vi "Detect edge angles.vi"(0 "Image filepath":path=path "E:/Algorithm/Geometric template matching/Images/Partially symmetric part/2.png", 1 "Auto ROI detect":bool=TRUE, 2 "Remove dust?":bool=TRUE, 3 "ROI parameters\nFeature":T5={"Step Size"=500, "r offset"=500, "Edge Options"={"Edge Polarity"=0, "Kernel Size"=5, "Width"=3, "Minimum Edge Strength"=120.0, "Interpolation Type"=enum."Bilinear Fixed", "Data Processing Method"=enum."Average"}, "Annulus\ndetails"={"Center X"=0, "Center Y"=0, "Inner Radius"=10, "Outer Radius"=4000, "Start Angle"=0.0, "End Angle"=0.0}} {"Edge Options"."Edge Polarity" items=["All Edges", "Rising Edges", "Falling Edges"]; "Edge Options"."Minimum Edge Strength" format="%.2f"; "Edge Options"."Width" step=2; "Edge Options"."Kernel Size" step=2; "Annulus\ndetails"."End Angle" min=-90.0 max=90.0 step=1.0 format="%.2f"; "Annulus\ndetails"."Start Angle" min=-90.0 max=90.0 step=1.0 format="%.2f"; "Annulus\ndetails"."Center X" scale=0.0..1024.0}, 4 "Image input?":bool, 5 "error in":errorcluster, 6 "Image in":T1, 7 "Overlay?":bool=TRUE, 8 "Dispose\nimage?":bool, 9 "Dust removal data":T7={"Dilate data"={"Operation"=enum."Erode", "Structuring Element"=[[1, 1, 1], [1, 1, 1], [1, 1, 1]], "Number of iterations (1)"=1, "Square/Hexa (Square)"=TRUE}, "Threshold data"={"Method (clustering)"=0, "Look For (Bright Objects)"=1, "Range"={"Lower value"=128.0, "Upper value"=255.0}, "Replace Value"=1.0}} {"Threshold data"."Look For (Bright Objects)" items=["Bright Objects", "Dark Objects"]; "Threshold data"."Method (clustering)" items=["clustering", "entropy", "metric", "moments", "inter-class variance"]}, 11 "BufferData":cluster{"Image Name":string}={"Image Name"="LearnTempImage"}) -> (10 "ROI parameters\nFeature out":T8 {"Edge Options"."Edge Polarity" items=["All Edges", "Rising Edges", "Falling Edges"]; "Edge Options"."Minimum Edge Strength" format="%.2f"; "Edge Options"."Width" step=2; "Edge Options"."Kernel Size" step=2; "Annulus\ndetails"."End Angle" min=-90.0 max=90.0 step=1.0 format="%.2f"; "Annulus\ndetails"."Start Angle" min=-90.0 max=90.0 step=1.0 format="%.2f"; "Annulus\ndetails"."Center X" scale=0.0..1024.0}, 14 "Output":T6, 16 "Image indicator":T1(plugin-control), 19 "error out":errorcluster)   [LabVIEW 2019]
uses:
  <vilib>/vision/Image Controls.llb/IMAQ Image.ctl
  <vilib>/vision/Measure.llb/Edge Options.ctl
  <vilib>/vision/Measure.llb/Edge Polarity.ctl
  <vilib>/Utility/file.llb/Write Delimited Spreadsheet (DBL).vi
  Controls/ROI parameters.ctl
panel:
  in  "Tab Control":enum32{"Display image", "Misc."}(tab)
  out "Output filepath":path
  in  "stop":bool
  out "Cycle time (in seconds)":dbl
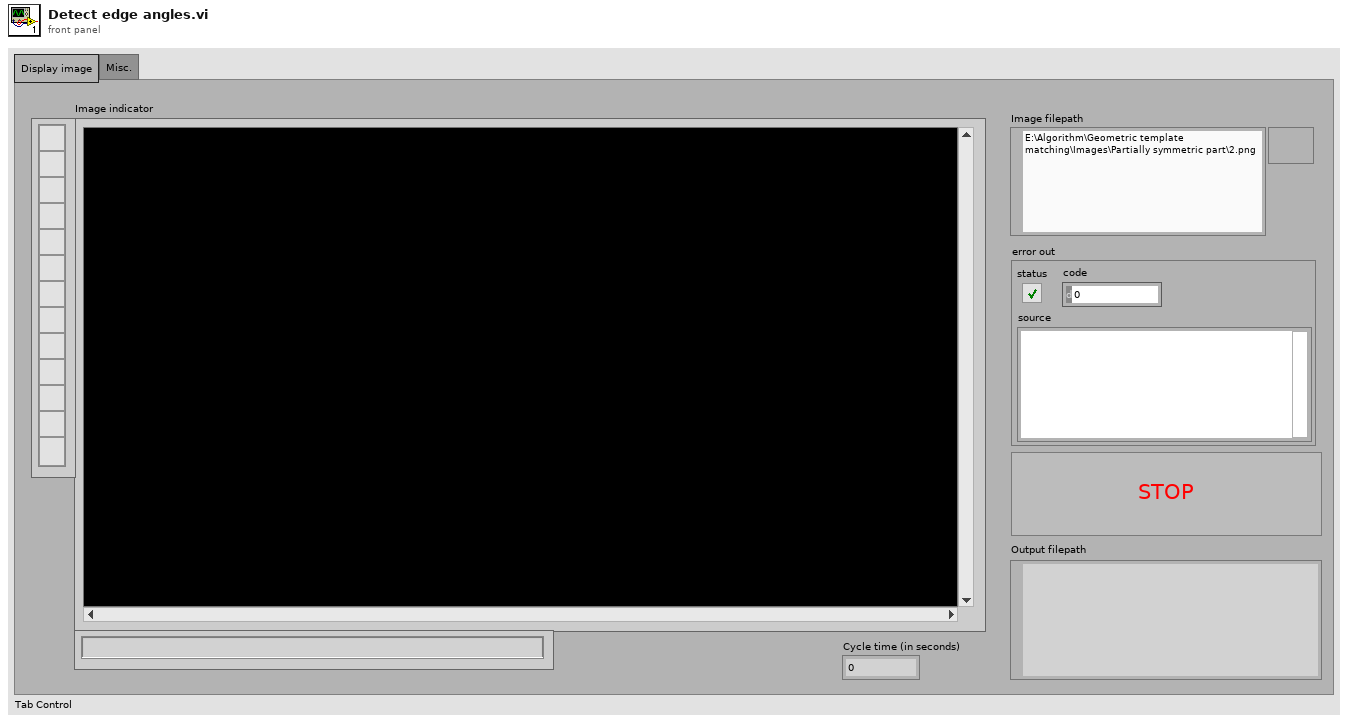
[diagram p1: front panel]
types:
  T1 = typedef "IMAQ Image.ctl" = refnum<image>
  T2 = typedef "Edge Options.ctl" = cluster{"Edge Polarity":T3, "Kernel Size":u32, "Width":u32, "Minimum Edge Strength":sgl, "Interpolation Type":enum32{"Zero Order", "Bilinear", "Quadratic", "Cubic", "Bilinear Fixed"}, "Data Processing Method":enum32{"Average", "Median"}}
  T3 = typedef "Edge Polarity.ctl" = u32
  T4 = typedef "IMAQ Circle" = cluster{"Center X":i32, "Center Y":i32, "Inner Radius":i32, "Outer Radius":i32, "Start Angle":dbl, "End Angle":dbl}
  T5 = cluster{"Step Size":u32, "r offset":u32, "Edge Options":T2, "Annulus\ndetails":T4}
  T6 = cluster{"Angle info":cluster{"Rising edge angles":cluster{"Edge angles":dbl[]}[], "Falling edge angles":cluster{"Edge angles":dbl[]}[]}, "Center":cluster{"X":sgl, "Y":sgl}}
  T7 = cluster{"Dilate data":cluster{"Operation":enum32{"AutoM", "Close", "Dilate", "Erode", "Gradient", "Gradient out", "Gradient in", "Hit miss", "Open", "PClose", "POpen", "Thick", "Thin"}, "Structuring Element":i32[][], "Number of iterations (1)":i32, "Square/Hexa (Square)":bool}, "Threshold data":cluster{"Method (clustering)":i32, "Look For (Bright Objects)":u32, "Range":cluster{"Lower value":sgl, "Upper value":sgl}, "Replace Value":sgl}}
  T8 = typedef "ROI parameters.ctl" = cluster{"Step Size":u32, "r offset":u32, "Edge Options":T2, "Annulus\ndetails":T4}
  T9 = cluster{"Rising edge angles":cluster{"Edge angles":dbl[]}[], "Falling edge angles":cluster{"Edge angles":dbl[]}[]}
  T10 = cluster{"Edges (Rising)":cluster{"Location":cluster{"X":sgl, "Y":sgl}[]}[], "Edges (Falling)":cluster{"Location":cluster{"X":sgl, "Y":sgl}[]}[], "ROI parameters\nFeature.Edge Options":T2}
  T11 = cluster{"Global Rectangle":i32[], "Contours":cluster{"Contour Type":u32, "ROI Type":u32, "Points":i32[]}[]}
  T12 = cluster{"Center":cluster{"X":sgl, "Y":sgl}, "Radius":dbl}
  T13 = cluster{"Edge ROI":cluster{"Global Rectangle":i32[], "Contours":cluster{"Contour Type":u32, "ROI Type":u32, "Points":i32[]}[]}, "Previous state":string, "Circle 1 detaiils":cluster{"Center":cluster{"X":sgl, "Y":sgl}, "Radius":dbl}, "Image indicator":refnum<vi>, "Image \narray":T1[], "Edge point location":cluster{"X":sgl, "Y":sgl}[], "Angles":sgl[], "Output filename":string, "Tick count (Start)":u32, "ROI parameters\nFeature":cluster{"Step Size":u32, "r offset":u32, "Edge Options":T2, "Annulus\ndetails":T4}, "Edge info":cluster{"Edges (Rising)":cluster{"Location":cluster{"X":sgl, "Y":sgl}[]}[], "Edges (Falling)":cluster{"Location":cluster{"X":sgl, "Y":sgl}[]}[], "ROI parameters\nFeature.Edge Options":T2}, "Angle info":cluster{"Rising edge angles":cluster{"Edge angles":dbl[]}[], "Falling edge angles":cluster{"Edge angles":dbl[]}[]}, "Dust removal data":cluster{"Dilate data":cluster{"Operation":enum32{"AutoM", "Close", "Dilate", "Erode", "Gradient", "Gradient out", "Gradient in", "Hit miss", "Open", "PClose", "POpen", "Thick", "Thin"}, "Structuring Element":i32[][], "Number of iterations (1)":i32, "Square/Hexa (Square)":bool}, "Threshold data":cluster{"Method (clustering)":i32, "Look For (Bright Objects)":u32, "Range":cluster{"Lower value":sgl, "Upper value":sgl}, "Replace Value":sgl}}, "Remove dust?":bool, "Auto ROI detect":bool, "Image size factor":dbl, "Image in":T1, "Overlay?":bool, "BufferData":cluster{"Image Name":string}}
  T14 = cluster{"Objects":u16, "Threshold":i32, "Reject Border":bool, "Fill Holes":bool, "Min Object Size":bool, "Min Size":i32, "Max Object Size":bool, "Max Size":i32, "Show Search Area":bool, "Show Center":bool, "Show Bounding Box":bool}
  T15 = typedef "ROI Descriptor" = cluster{"Global Rectangle":i32[], "Contours":cluster{"ID":enum32{"External", "Internal"}, "Type":u32, "Coordinates":i32[]}[]}
  T16 = cluster{"Object Center":cluster{"X":sgl, "Y":sgl}, "Bounding Box":cluster{"X Left":i32, "Y Top":i32, "X Right":i32, "Y Bottom":i32}, "Area":sgl, "Orientation":sgl, "Aspect Ratio":sgl, "Nb Holes":i32}[]
  T17 = cluster{"Object Center":cluster{"X":sgl, "Y":sgl}, "Bounding Box":cluster{"X Left":i32, "Y Top":i32, "X Right":i32, "Y Bottom":i32}, "Area":sgl, "Orientation":sgl, "Aspect Ratio":sgl, "Nb Holes":i32}
  T18 = cluster{"Location":cluster{"X":sgl, "Y":sgl}[]}[]
  T19 = typedef "Image Type" = u32
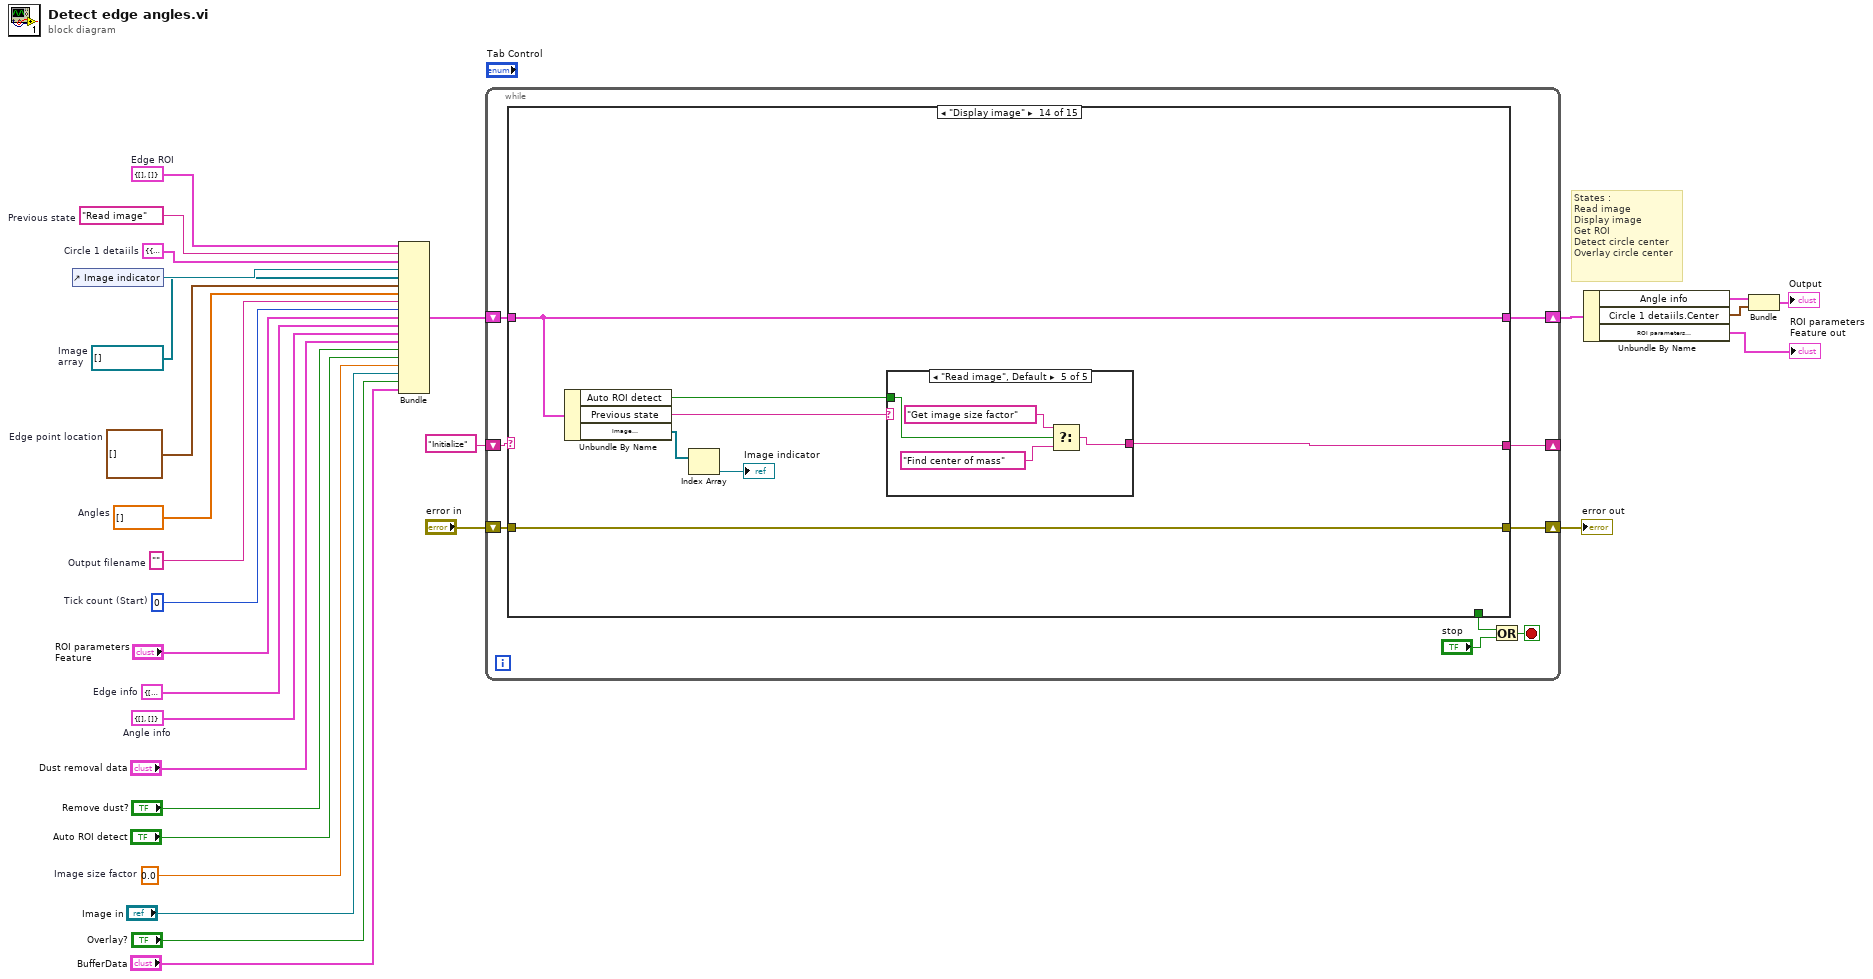
[diagram p0: block diagram]
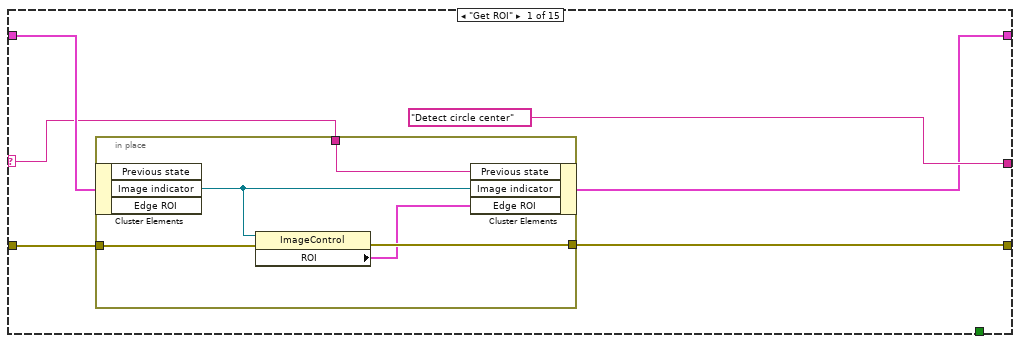
[diagram p2: hidden frame]
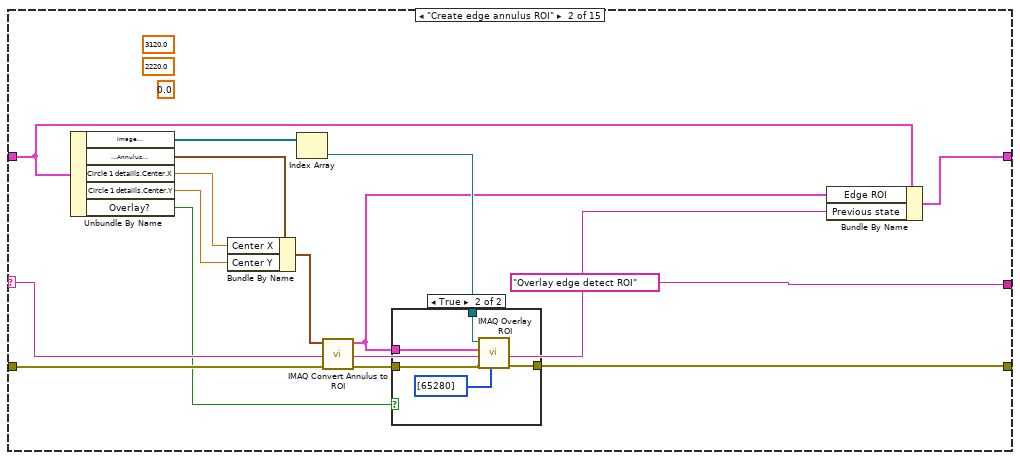
[diagram p3: hidden frame]
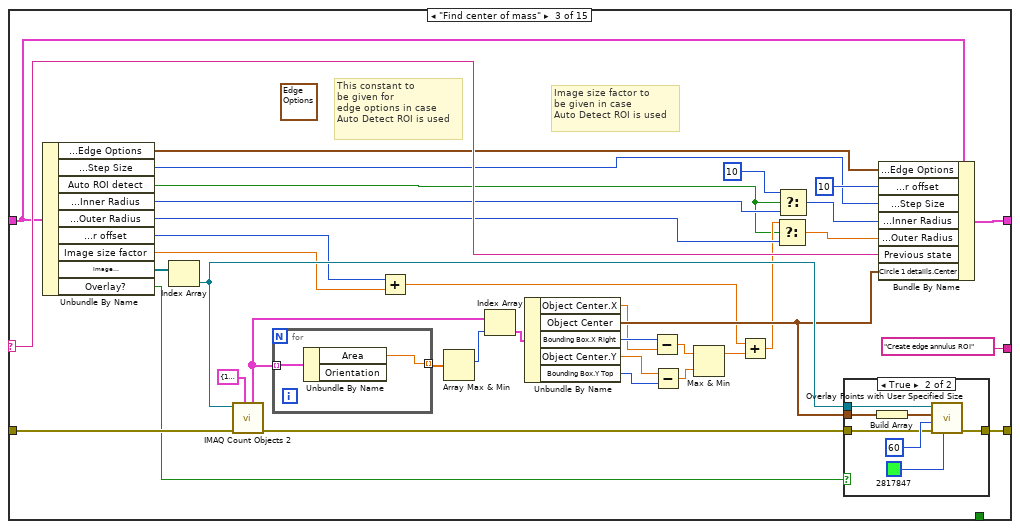
[diagram p5: hidden frame]
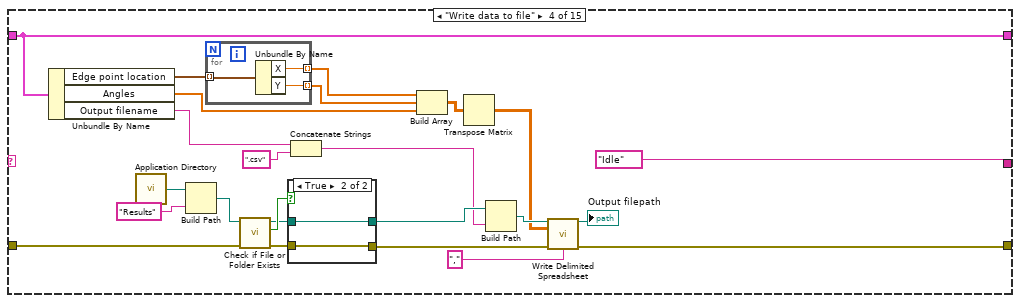
[diagram p7: hidden frame]
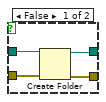
[diagram p8: hidden frame]
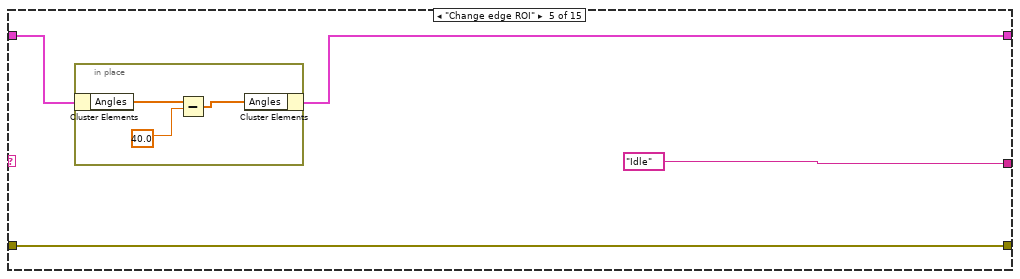
[diagram p9: hidden frame]
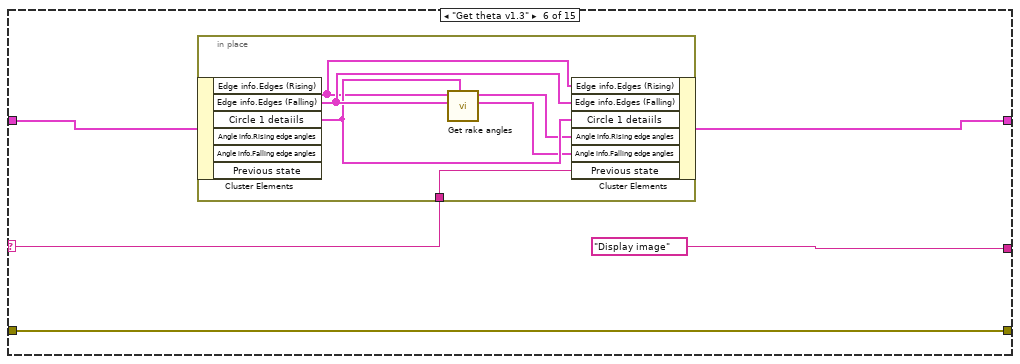
[diagram p10: hidden frame]
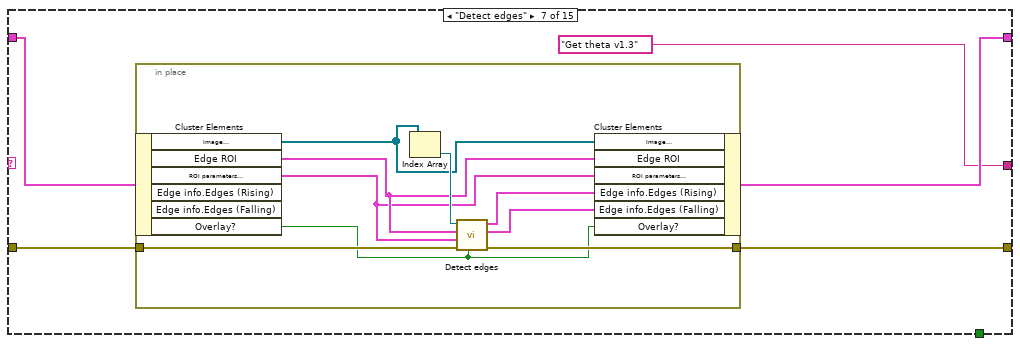
[diagram p11: hidden frame]
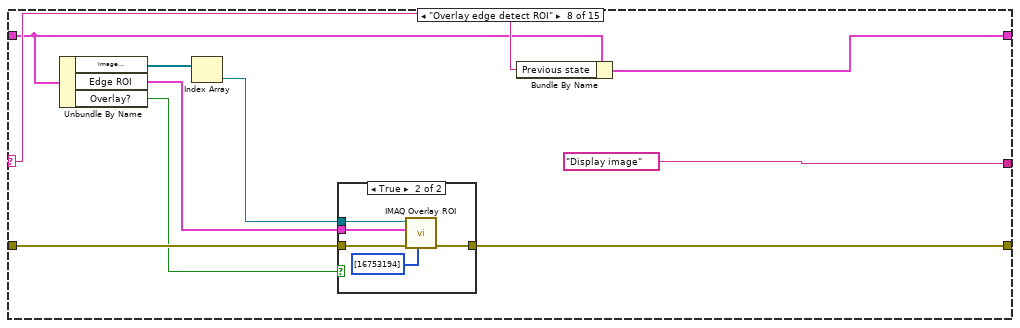
[diagram p12: hidden frame]
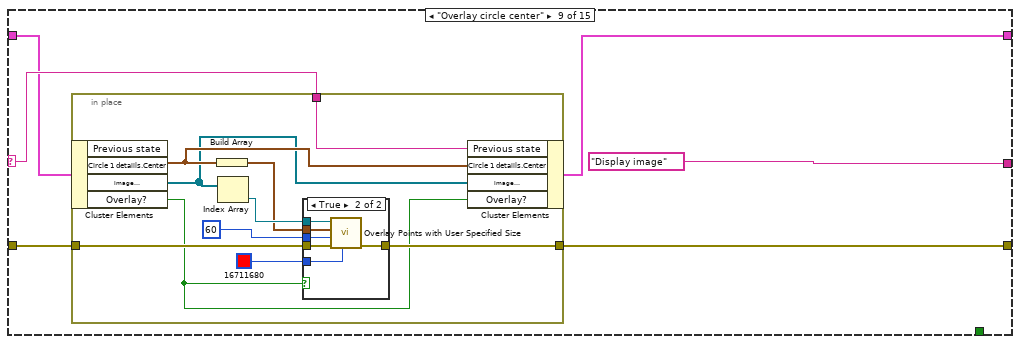
[diagram p14: hidden frame]
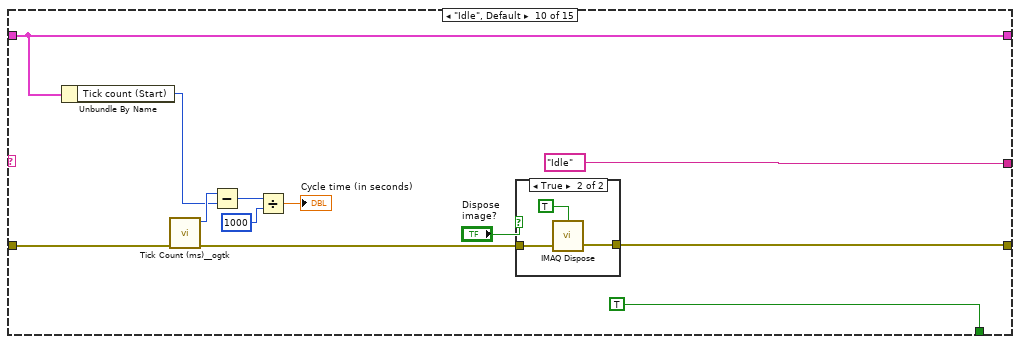
[diagram p16: hidden frame]
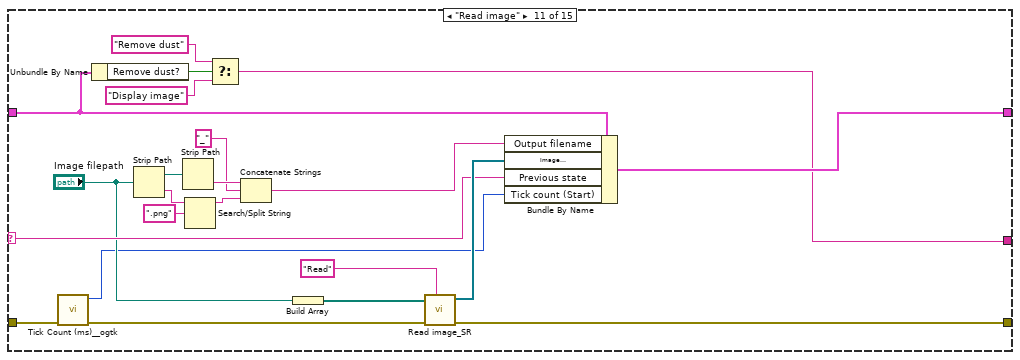
[diagram p18: hidden frame]
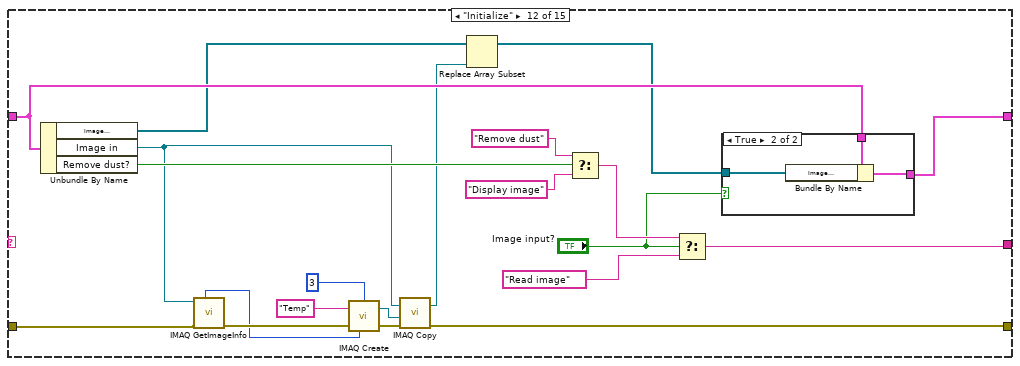
[diagram p19: hidden frame]
diagram:
  w6 = 0.0  # Image size factor
  w13 = T9 {"Rising edge angles"=[], "Falling edge angles"=[]}  # Angle info
  w14 = T10 {"Edges (Rising)"=[], "Edges (Falling)"=[], "ROI parameters\nFeature.Edge Options"={"Edge Polarity"=0, "Kernel Size"=3, "Width"=3, "Minimum Edge Strength"=10.0, "Interpolation Type"=enum."Bilinear Fixed", "Data Processing Method"=enum."Average"}}  # Edge info
  w18 = ""  # Output filename
  w17 = u32 0  # Tick count (Start)
  w19 = sgl[] []  # Angles
  w20 = cluster{"X":sgl, "Y":sgl}[] []  # Edge point location
  w21 = T11 {"Global Rectangle"=[], "Contours"=[]}  # Edge ROI
  w22 = "Read image"  # Previous state
  w24 = T12 {"Center"={"X"=0.0, "Y"=0.0}, "Radius"=0.0}  # Circle 1 detaiils
  w27 = T1[] []  # Image  array
  # "States :\nRead image\nDisplay image\nGet ROI\nDetect circle center\nOverlay circle center"
  n1 = control-ref of="Image indicator"() -> (w28:refnum<vi>)
  n2 = Bundle("Edge ROI"=w21, "Previous state"=w22, "Circle 1 detaiils"=w24, "Image indicator"=w28, "Image \narray"=w27, "Edge point location"=w20, "Angles"=w19, "Output filename"=w18, "Tick count (Start)"=w17, "ROI parameters\nFeature"="ROI parameters\nFeature", "Edge info"=w14, "Angle info"=w13, "Dust removal data"="Dust removal data", "Remove dust?"="Remove dust?", "Auto ROI detect"="Auto ROI detect", "Image size factor"=w6, "Image in"="Image in", "Overlay?"="Overlay?", "BufferData"="BufferData") -> (w26:T13)  [unwired: 1 in]
  n3 = while {
    shift-right: [w29] -> w16
    shift-left: w26 -> [w36]
    shift-right: [w33] -> _
    shift-left: "Initialize" ("Combo Box") -> [w37]
    shift-right: [w34] -> w23
    shift-left: "error in" -> [w35]
    stop <- w30 stop-if-true
    n4 = case shown="\"Display image\"" w37 {
      selector: w37 -> [w39 w62 w103 _ _ w156 _ w184 w199 _ w255 _ _ _ _]
      tunnel: w36 -> [w41 w63 w102 w131 w151 w159 w169 w183 w198 w228 w241 w272 w285 w298 w313]
      tunnel: w35 -> [w43 w60 w100 w129 w152 w160 w171 w190 w202 w227 w244 w261 w287 w300 w315]
      tunnel: [w42 w53 w105 w128 w152 w160 w170 w189 w201 w229 w257 w269 w286 w300 w314] -> w34
      tunnel: ["Detect circle center" ("Combo Box") "Overlay edge detect ROI" ("Combo Box") "Create edge annulus ROI" ("Combo Box") "Idle" ("Combo Box") "Idle" ("Combo Box") "Display image" ("Combo Box") "Get theta v1.3" ("Combo Box") "Display image" ("Combo Box") "Display image" ("Combo Box") "Idle" ("Combo Box") w237 w273 "Display image" ("Combo Box") w297 "Find center of mass" ("Combo Box")] -> w33
      tunnel: [_ _ _ _ _ _ _ _ _ TRUE _ _ _ _ _] -> w31
      tunnel: [w38 w56 w101 w131 w150 w158 w168 w182 w197 w228 w254 w270 w284 w298 w312] -> w29
      frame "Get ROI" {
        n5 = in-place {
          in-place-border: w43 -> [w48]
          in-place-border: [w47] -> w42
          in-place-border: w39 -> [w44]
          n6 = in-place-cluster #1(w41) -> ("Image indicator"=w46:refnum<vi>)  [unwired: 2 out]
          n7 = property class="ImageControl"(reference=w46, error in=w48) -> (error out=w47:errorcluster, "ROI"=w45:T11)  [unwired: 1 out]
          n8 = in-place-cluster #1("Previous state"=w44, "Image indicator"=w46, "Edge ROI"=w45) -> (w38:T13)
        }
      }
      frame "Create edge annulus ROI" {
        (unwired) sgl 0.0 ("element")
        (unwired) sgl 2220.0 ("y")
        (unwired) sgl 3120.0 ("y")
        n9 = Unbundle By Name(w63) -> ("Image \narray"=w52:T1[], "ROI parameters\nFeature.Annulus\ndetails"=w55:T4, "Circle 1 detaiils.Center.X"=w59:sgl, "Circle 1 detaiils.Center.Y"=w58:sgl, "Overlay?"=w49:bool)
        n10 = Bundle By Name(cluster=w55, "Center X"=w59, "Center Y"=w58) -> (w57:T4)
        n11 = Index Array(array=w52) -> (element=w51:T1)  [unwired: 1 in]
        n12 = call "IMAQ Convert Annulus to ROI"("error in (no error)"=w60, "Annulus"=w57) -> ("error out"=w54:errorcluster, "ROI Descriptor"=w50:T15)  [unwired: 7 in]
        n13 = case shown="True" w49 {
          tunnel: w54 -> [w64 w69]
          tunnel: [w64 w68] -> w53
          tunnel: w51 -> [_ w67]
          tunnel: w50 -> [_ w66]
          frame False {
          }
          frame True {
            n14 = call "IMAQ Overlay ROI"("Colors (Green)"=u32[] [65280], "error in (no error)"=w69, "ROI Descriptor"=w66, "Image"=w67) -> ("error out"=w68:errorcluster)  [unwired: 6 in, 1 out]
          }
        }
        n15 = Bundle By Name(cluster=w63, "Edge ROI"=w50, "Previous state"=w62) -> (w56:T13)
      }
      frame "Find center of mass" {
        (unwired) T2 {"Edge Polarity"=0, "Kernel Size"=7, "Width"=5, "Minimum Edge Strength"=100.0, "Interpolation Type"=enum."Bilinear Fixed", "Data Processing Method"=enum."Average"} ("ROI parameters\nFeature.Edge Options")
        # "This constant to\nbe given for\nedge options in case\nAuto Detect ROI is used"
        # "Image size factor to\nbe given in case\nAuto Detect ROI is used"
        n16 = Unbundle By Name(w102) -> ("ROI parameters\nFeature.Edge Options"=w71:T2, "ROI parameters\nFeature.Step Size"=w72:u32, "Auto ROI detect"=w73:bool, "ROI parameters\nFeature.Annulus\ndetails.Inner Radius"=w89:i32, "ROI parameters\nFeature.Annulus\ndetails.Outer Radius"=w88:i32, "ROI parameters\nFeature.r offset"=w83:u32, "Image size factor"=w80:dbl, "Image \narray"=w84:T1[], "Overlay?"=w70:bool)
        n17 = Index Array(array=w84) -> (element=w98:T1)  [unwired: 1 in]
        n18 = call "IMAQ Count Objects 2"("Settings"=T14 {"Objects"=1, "Threshold"=128, "Reject Border"=FALSE, "Fill Holes"=FALSE, "Min Object Size"=FALSE, "Min Size"=3, "Max Object Size"=FALSE, "Max Size"=100, "Show Search Area"=FALSE, "Show Center"=FALSE, "Show Bounding Box"=FALSE}, "error in (no error)"=w100, "Image"=w98) -> ("error out"=w99:errorcluster, "Objects"=w95:T16)  [unwired: 4 in, 3 out]
        n19 = for {
          tunnel: w95 -> [w115] mode=indexing
          tunnel: [w114] -> w96 mode=indexing
          n20 = Unbundle By Name(w115) -> ("Area"=w114:sgl)  [unwired: 1 out]
        }
        n21 = Add(x=w83, y=w80) -> (x+y=w81:dbl)
        n22 = Array Max & Min(array=w96) -> (max index (indices)=w94:i32)  [unwired: 3 out]
        n23 = Index Array(array=w95, index=w94) -> (element=w93:T17)
        n24 = Unbundle By Name(w93) -> ("Object Center.X"=w90:sgl, "Object Center"=w92:cluster{"X":sgl, "Y":sgl}, "Bounding Box.X Right"=w91:i32, "Object Center.Y"=w79:sgl, "Bounding Box.Y Top"=w78:i32)
        n25 = Subtract(x=w91, y=w90) -> (x-y=w77:sgl)
        n26 = Subtract(x=w79, y=w78) -> (x-y=w76:sgl)
        n27 = Max & Min(x=w77, y=w76) -> (max(x,y)=w75:sgl)  [unwired: 1 out]
        n28 = Add(x=w81, y=w75) -> (x+y=w87:dbl)
        n29 = Select(t=w87, s=w73, f=w88) -> (s? t:f=w82:dbl)
        n30 = Select(t=10, s=w73, f=w89) -> (s? t:f=w85:i32)
        n31 = case shown="True" w70 {
          tunnel: [w106 w113] -> w105
          tunnel: w99 -> [w106 w110]
          tunnel: w98 -> [_ w109]
          tunnel: w92 -> [_ w108]
          frame False {
          }
          frame True {
            n32 = Build Array(w108) -> (w107:cluster{"X":sgl, "Y":sgl}[])
            n33 = call "Overlay Points with User Specified Size.vi"("Color"=u32 2817847, "error in"=w110, "Point Diameter (5)"=u32 60, "Points"=w107, "Image In"=w109) -> ("error out"=w113:errorcluster)  [unwired: 5 in, 1 out]
          }
        }
        n34 = Bundle By Name(cluster=w102, "ROI parameters\nFeature.Edge Options"=w71, "ROI parameters\nFeature.r offset"=u32 10 ("ROI parameters\nFeature.r offset"), "ROI parameters\nFeature.Step Size"=w72, "ROI parameters\nFeature.Annulus\ndetails.Inner Radius"=w85, "ROI parameters\nFeature.Annulus\ndetails.Outer Radius"=w82, "Previous state"=w103, "Circle 1 detaiils.Center"=w92) -> (w101:T13)
      }
      frame "Write data to file" {
        n35 = Unbundle By Name(w131) -> ("Edge point location"=w118:cluster{"X":sgl, "Y":sgl}[], "Angles"=w126:sgl[], "Output filename"=w125:string)
        n36 = call <vilib>:"Application Directory.vi"() -> ("Application Directory"=w132:path)
        n37 = Build Path(base path=w132, name or relative path="Results") -> (appended path=w135:path)
        n38 = for {
          tunnel: w118 -> [w142] mode=indexing
          tunnel: [w141] -> w117 mode=indexing
          tunnel: [w140] -> w116 mode=indexing
          n39 = Unbundle By Name(w142) -> ("X"=w141:sgl, "Y"=w140:sgl)
        }
        n40 = call <vilib>:"Check if File or Folder Exists.vi"("error in (no error)"=w129, "path"=w135) -> ("error out"=w134:errorcluster, "file or folder exists?"=w137:bool, "dup path"=w136:path)  [unwired: 7 in]
        n41 = case shown="True" w137 {
          tunnel: w134 -> [w146 w148]
          tunnel: w136 -> [w145 w147]
          tunnel: [w144 w148] -> w138
          tunnel: [w143 w147] -> w139
          frame False {
            n42 = Create Folder(path (use dialog)=w145, error in=w146) -> (created path=w143:path, error out=w144:errorcluster)  [unwired: 1 in, 1 out]
          }
          frame True {
          }
        }
        n43 = Concatenate Strings(w125, ".csv" ("string")) -> (w123:string)
        n44 = Build Array(w117, w116, w126) -> (w121:sgl[][])
        n45 = Transpose Matrix(1:w121) -> (0:w120:dbl[][])
        n46 = Build Path(base path=w139, name or relative path=w123) -> (appended path=w130:path)
        n47 = call-poly <vilib>:"Write Delimited Spreadsheet.vi"("file path (dialog if empty)"=w130, "2D data"=w120, "error in (no error)"=w138, "delimiter (\\t)"="," ("delimiter (\\t)")) -> ("new file path (Not A Path if cancelled)"=→"Output filepath":path, "error out"=w128:errorcluster)  [unwired: 10 in]
      }
      frame "Change edge ROI" {
        n48 = in-place {
          n49 = in-place-cluster #2(w151) -> ("Angles"=w155:sgl[])
          n50 = Subtract(x=w155, y=sgl 40.0) -> (x-y=w153:sgl[])
          n51 = in-place-cluster #2("Angles"=w153) -> (w150:T13)
        }
      }
      frame "Get theta v1.3" {
        n52 = in-place {
          in-place-border: w156 -> [w162]
          n53 = in-place-cluster #3(w159) -> ("Edge info.Edges (Rising)"=w161:T18, "Edge info.Edges (Falling)"=w166:T18, "Circle 1 detaiils"=w165:T12)  [unwired: 3 out]
          n54 = call "Get rake angles.vi"("Circle details"=w165, "Edges (Falling)"=w166, "Edges (Rising)"=w161) -> ("Falling edge angles"=w163:cluster{"Edge angles":dbl[]}[], "Rising edge angles"=w164:cluster{"Edge angles":dbl[]}[])  [unwired: 7 in]
          n55 = in-place-cluster #3("Edge info.Edges (Rising)"=w161, "Edge info.Edges (Falling)"=w166, "Circle 1 detaiils"=w165, "Angle info.Rising edge angles"=w164, "Angle info.Falling edge angles"=w163, "Previous state"=w162) -> (w158:T13)
        }
      }
      frame "Detect edges" {
        n56 = in-place {
          in-place-border: w171 -> [w180]
          in-place-border: [w179] -> w170
          n57 = in-place-cluster #4(w169) -> ("Image \narray"=w177:T1[], "Edge ROI"=w176:T11, "ROI parameters\nFeature"=w173:T5, "Overlay?"=w172:bool)  [unwired: 2 out]
          n58 = Index Array(array=w177) -> (element=w178:T1)  [unwired: 1 in]
          n59 = call "Detect edges.vi"("Overlay?"=w172, "error in (no error)"=w180, "ROI parameters\nFeature"=w173, "ROI"=w176, "Image"=w178) -> ("error out"=w179:errorcluster, "Edges (Falling)"=w174:T18, "Edges (Rsiing)"=w175:T18)  [unwired: 3 in, 1 out]
          n60 = in-place-cluster #4("Image \narray"=w177, "Edge ROI"=w176, "ROI parameters\nFeature"=w173, "Edge info.Edges (Rising)"=w175, "Edge info.Edges (Falling)"=w174, "Overlay?"=w172) -> (w168:T13)
        }
      }
      frame "Overlay edge detect ROI" {
        n61 = Unbundle By Name(w183) -> ("Image \narray"=w188:T1[], "Edge ROI"=w186:T11, "Overlay?"=w181:bool)
        n62 = Index Array(array=w188) -> (element=w187:T1)  [unwired: 1 in]
        n63 = case shown="True" w181 {
          tunnel: w190 -> [w191 w196]
          tunnel: [w191 w195] -> w189
          tunnel: w187 -> [_ w194]
          tunnel: w186 -> [_ w193]
          frame False {
          }
          frame True {
            n64 = call "IMAQ Overlay ROI"("Colors (Green)"=u32[] [16753194], "error in (no error)"=w196, "ROI Descriptor"=w193, "Image"=w194) -> ("error out"=w195:errorcluster)  [unwired: 6 in, 1 out]
          }
        }
        n65 = Bundle By Name(cluster=w183, "Previous state"=w184) -> (w182:T13)
      }
      frame "Overlay circle center" {
        n66 = in-place {
          in-place-border: w202 -> [w212]
          in-place-border: [w211] -> w201
          in-place-border: w199 -> [w204]
          n67 = in-place-cluster #5(w198) -> ("Circle 1 detaiils.Center"=w206:cluster{"X":sgl, "Y":sgl}, "Image \narray"=w205:T1[], "Overlay?"=w203:bool)  [unwired: 1 out]
          n68 = Build Array(w206) -> (w209:cluster{"X":sgl, "Y":sgl}[])
          n69 = Index Array(array=w205) -> (element=w210:T1)  [unwired: 1 in]
          n70 = case shown="True" w203 {
            tunnel: w212 -> [w213 w219]
            tunnel: [w213 w218] -> w211
            tunnel: w210 -> [_ w217]
            tunnel: w209 -> [_ w216]
            tunnel: u32 60 ("Point Diameter (5)") -> [_ w215]
            tunnel: u32 16711680 ("Color") -> [_ w214]
            frame False {
            }
            frame True {
              n71 = call "Overlay Points with User Specified Size.vi"("Color"=w214, "error in"=w219, "Point Diameter (5)"=w215, "Points"=w216, "Image In"=w217) -> ("error out"=w218:errorcluster)  [unwired: 5 in, 1 out]
            }
          }
          n72 = in-place-cluster #5("Previous state"=w204, "Circle 1 detaiils.Center"=w206, "Image \narray"=w205, "Overlay?"=w203) -> (w197:T13)
        }
      }
      frame "Idle", Default {
        n73 = Unbundle By Name(w228) -> ("Tick count (Start)"=w224:u32)
        n74 = call <userlib>:"Tick Count (ms)__ogtk.vi"("error in (no error)"=w227) -> ("error out"=w226:errorcluster, "millisecond timer value"=w225:u32)  [unwired: 9 in]
        n75 = Subtract(x=w225, y=w224) -> (x-y=w223:u32)
        n76 = Divide(x=w223, y=u32 1000) -> (x/y=→"Cycle time (in seconds)":dbl)
        n77 = case shown="True" "Dispose\nimage?" {
          tunnel: [w232 w235] -> w229
          tunnel: w226 -> [w232 w234]
          frame False {
          }
          frame True {
            n78 = call "IMAQ Dispose"("All Images? (No)"=TRUE, "error in (no error)"=w234) -> ("error out"=w235:errorcluster)  [unwired: 4 in]
          }
        }
      }
      frame "Read image" {
        n79 = call <userlib>:"Tick Count (ms)__ogtk.vi"("error in (no error)"=w244) -> ("error out"=w243:errorcluster, "millisecond timer value"=w242:u32)  [unwired: 9 in]
        n80 = Unbundle By Name(w241) -> ("Remove dust?"=w240:bool)
        n81 = Strip Path(path="Image filepath") -> (stripped path=w252:path, name=w248:string)
        n82 = Strip Path(path=w252) -> (name=w251:string)  [unwired: 1 out]
        n83 = Search/Split String(string=w248, search string/char (-)=".png") -> (substring before match=w246:string)  [unwired: 1 in, 2 out]
        n84 = Select(t="Remove dust", s=w240, f="Display image") -> (s? t:f=w237:string)
        n85 = Concatenate Strings(w251, "_" ("string"), w246) -> (w245:string)
        n86 = Build Array("Image filepath") -> (w253:path[])
        n87 = call "Read image_SR.vi"("Concatenating string"="Read", "error in (no error)"=w243, "Image filepath array"=w253) -> ("error out"=w257:errorcluster, "Image \narray"=w256:T1[])  [unwired: 6 in, 1 out]
        n88 = Bundle By Name(cluster=w241, "Output filename"=w245, "Image \narray"=w256, "Previous state"=w255, "Tick count (Start)"=w242) -> (w254:T13)
      }
      frame "Initialize" {
        n89 = Unbundle By Name(w272) -> ("Image \narray"=w264:T1[], "Image in"=w259:T1, "Remove dust?"=w274:bool)
        n90 = call "IMAQ GetImageInfo"("error in (no error)"=w261, "Image"=w259) -> ("error out"=w260:errorcluster, "Image Type"=w258:T19)  [unwired: 2 in, 6 out]
        n91 = call "IMAQ Create"("Border Size"=3, "Image Name"="Temp", "Image Type"=w258, "error in (no error)"=w260) -> ("New Image"=w265:T1, "error out"=w268:errorcluster)  [unwired: 1 in]
        n92 = call "IMAQ Copy"("error in (no error)"=w268, "Image Dst"=w265, "Image Src"=w259) -> ("error out"=w269:errorcluster, "Image Dst Out"=w263:T1)  [unwired: 3 in]
        n93 = Replace Array Subset(array=w264, new element=w263) -> (w262:T1[])  [unwired: 1 in]
        n94 = Select(t="Remove dust", s=w274, f="Display image") -> (s? t:f=w278:string)
        n95 = Select(t=w278, s="Image input?", f="Read image" ("Combo Box")) -> (s? t:f=w273:string)
        n96 = case shown="True" "Image input?" {
          tunnel: w272 -> [w279 w282]
          tunnel: w262 -> [_ w281]
          tunnel: [w279 w280] -> w270
          frame False {
          }
          frame True {
            n97 = Bundle By Name(cluster=w282, "Image \narray"=w281) -> (w280:T13)
          }
        }
      }
      frame "Remove dust" {
        n98 = in-place {
          in-place-border: w287 -> [w295]
          in-place-border: [w294] -> w286
          n99 = in-place-cluster #6(w285) -> ("Image \narray"=w291:T1[], "Dust removal data"=w292:T7)
          n100 = Index Array(array=w291) -> (element=w293:T1)  [unwired: 1 in]
          n101 = call "RemoveDust.vi"("error in (no error)"=w295, "Dust removal data"=w292, "Image in"=w293) -> ("error out"=w294:errorcluster, "Image out"=w290:T1)  [unwired: 7 in]
          n102 = Replace Array Subset(array=w291, new element=w290, index=0) -> (w289:T1[])
          n103 = in-place-cluster #6("Image \narray"=w289, "Dust removal data"=w292) -> (w284:T13)
        }
      }
      frame "Display image" {
        n104 = Unbundle By Name(w298) -> ("Auto ROI detect"=w296:bool, "Previous state"=w299:string, "Image \narray"=w301:T1[])
        n105 = Index Array(array=w301) -> (element=→"Image indicator":T1)  [unwired: 1 in]
        n106 = case shown="\"Read image\", Default" w299 {
          tunnel: ["Create edge annulus ROI" ("Combo Box") "Detect edges" ("Combo Box") "Idle" ("Combo Box") "Find r" ("Combo Box") w307] -> w297
          tunnel: w296 -> [_ _ _ _ w310]
          frame "Overlay circle center" {
          }
          frame "Overlay edge detect ROI" {
          }
          frame "Get theta v1.3" {
          }
          frame "Detect edge points" {
          }
          frame "Read image", Default {
            n107 = Select(t="Get image size factor" ("Combo Box"), s=w310, f="Find center of mass" ("Combo Box")) -> (s? t:f=w307:string)
          }
        }
      }
      frame "Get image size factor" {
        n108 = in-place {
          in-place-border: w315 -> [w324]
          in-place-border: [w323] -> w314
          # "Put based on  maximum\npossible image size"
          n109 = in-place-cluster #7(w313) -> ("Image \narray"=w317:T1[])  [unwired: 1 out]
          n110 = Index Array(array=w317) -> (element=w322:T1)  [unwired: 1 in]
          n111 = call "IMAQ GetImageSize"("Image"=w322, "error in (no error)"=w324) -> ("Y Resolution"=w320:i32, "X Resolution"=w321:i32, "error out"=w323:errorcluster)  [unwired: 2 in]
          n112 = Add(x=w321, y=w320) -> (x+y=w319:i32)
          n113 = Divide(x=w319, y=350) -> (x/y=w316:dbl)
          n114 = in-place-cluster #7("Image size factor"=w316, "Image \narray"=w317) -> (w312:T13)
        }
      }
    }
    n115 = Or(x=w31, y="stop") -> (x .or. y?=w30:bool)
  }
  "error out" <- w23
  n116 = Unbundle By Name(w16) -> ("Angle info"=w12:T9, "Circle 1 detaiils.Center"=w11:cluster{"X":sgl, "Y":sgl}, "ROI parameters\nFeature"=→"ROI parameters\nFeature out":T5)
  n117 = Bundle("Angle info"=w12, "Center"=w11) -> (→"Output":T6)  [unwired: 1 in]
